vi "DefaultFromINI.vi"(8 "error in (no error)":errorcluster, 11 "NhRegenGridSim":refnum<class "NHRGridSim.lvclass">) -> (0 "error out":errorcluster, 3 "NhRegenGridSim":refnum<class "NHRGridSim.lvclass">)   [LabVIEW 2018, in "AcPwrPlugins.lvlib" / "NHRGridSim.lvclass"]
doc: "This VI reads the properties from the INI file and puts them into the LabVIEW class for further use."
uses:
  NHRGridSim.lvclass
  C:/Program Files (x86)/National Instruments/LabVIEW 2018/user.lib/NIST/BaseClasses/BasePlugin_class/BasePlugin.lvclass
  C:/Projects/SmartGrid/ICDAS/NistPluggableModules/AcPwr/AcPwrPlugins/AcPwrBaseClass/AcPwrBase.lvclass
  Measurements.ctl
  TypeDefs/MeasurementType.ctl
  TypeDefs/Device(s)Settings.ctl
  TypeDefs/Modules.ctl
  <userlib>/NIST/BaseClasses/BasePlugin_class/BasePlugin.lvclass/BasePlugin.ctl
  <userlib>/NIST/BaseClasses/BasePlugin_class/Accessors/Read PluginIniFilePath.vi
  AcPwrBaseClass/AcPwrBase.lvclass
  <vilib>/Utility/config.llb/NI_LVConfig.lvlib
  TestClass/Test.lvclass
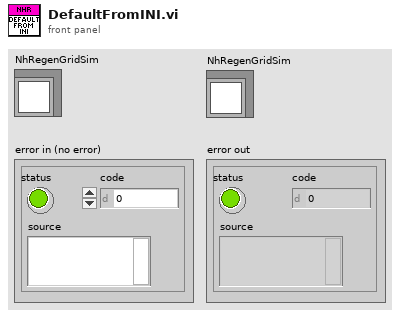
[diagram p1: front panel]
types:
  T1 = typedef "AcPwrPlugins.lvlib/NHRGridSim.lvclass/Device(s)Settings.ctl" = cluster{"MeasName":string, "Modules":T2}
  T2 = typedef "AcPwrPlugins.lvlib/NHRGridSim.lvclass/Modules.ctl" = cluster{"Measurement":cluster{"ApertureLength (s)":dbl, "NumberOfSamples":u32}, "Ranges":cluster{"Irange (A)":dbl, "Vrange (V)":dbl}, "Mode":u8, "Handle":string, "FreqOut (Hz)":dbl, "Connected":bool, "btnIdQuery":bool, "btnReset":bool, "Initialize Timeout ( ms)":u32, "Phase (0: All)":i32, "WatchDog":cluster{"Enable WatchDog":bool, "Robust WatchDog":bool, "Watchdog Interval (s)":dbl}, "Safety Limits":cluster{"Min Voltage (V)":dbl, "Min Voltage Time (s)":dbl, "Max Voltage (V)":dbl, "MaxVoltage Time (s)":dbl, "Max Source Amps (A)":dbl, "Max Source Amps Time (s)":dbl, "Max Sink Amps (A)":dbl, "Max Sink Amps Time (s)":dbl, "Max Source Power (W)":dbl, "Max Source Power Time (s)":dbl, "Max Sink Power (W)":dbl, "Max Sink Power Time (s)":dbl, "Peak Voltage (V)":dbl, "Peak Voltage Enable":bool, "Peak Amps (A)":dbl, "Peak Amps Enable":bool}, "Phases":cluster{"Pout (W)":dbl, "Iout (A)":dbl, "PhaseAngle":dbl, "Vout (V)":dbl, "Phase Name":string}[], "Regulation Gain":dbl, "ChangeOntheFly":bool, "Synchronize Output \nto Phase":bool, "Slew Rate":cluster{"Voltage Slew (Volts/s)":dbl, "Phase Angle (Degrees/s)":dbl}}[]
  T3 = typedef "AcPwrPlugins.lvlib/NHRGridSim.lvclass/Measurements.ctl" = cluster{"Handle":string, "Name":string, "Enabled ":bool, "Measurement Value":dbl, "Phase ":i32, "Measurement Type ":T4}[]
  T4 = typedef "AcPwrPlugins.lvlib/NHRGridSim.lvclass/MeasurementType.ctl" = enum16{"Average Current", "Average Voltage"}
  T5 = typedef "NI_LVConfig.lvlib/Config Data RefNum.ctl" = refnum<k1>
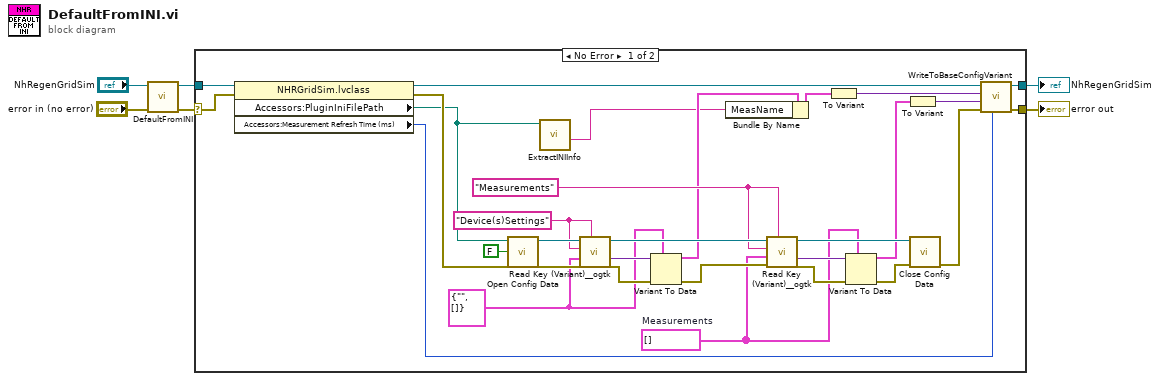
[diagram p0: block diagram]
diagram:
  n1 = call-parent "DefaultFromINI.vi"("error in (no error)"="error in (no error)", "AcPwrBase"="NhRegenGridSim") -> ("error out"=w1:errorcluster, "AcPwrBase"=w4:refnum<class "NHRGridSim.lvclass">)  [unwired: 8 in]
  n2 = case shown="No Error" w1 {
    selector: w1 -> [w29 w37]
    tunnel: w4 -> [w36 w38]
    tunnel: [w12 w38] -> w6
    tunnel: [w18 w37] -> w5
    frame No Error {
      w10 = T1 {"MeasName"="", "Modules"=[]} ("Device(s)Settings")
      w20 = T3 []  # Measurements
      w21 = "Measurements" ("section")
      w30 = "Device(s)Settings" ("section")
      n3 = property class="NHRGridSim.lvclass"(reference=w36, error in=w29) -> (reference out=w13:refnum<class "NHRGridSim.lvclass">, error out=w28:errorcluster, "Accessors:PluginIniFilePath"=w8:path, "Accessors:Measurement Refresh Time (ms)"=w11:u32)
      n4 = call <vilib>:"Open Config Data.vi"("error in (no error)"=w28, "create file if necessary (T)"=FALSE, "configuration file path"=w8) -> ("error out"=w33:errorcluster, "refnum"=w34:T5)  [unwired: 6 in, 1 out]
      n5 = call "ExtractINIInfo.vi"("INI File Path"=w8) -> ("Plugin Name"=w7:string)  [unwired: 8 in, 2 out]
      n6 = call <userlib>:"Read Key (Variant)__ogtk.vi"("section"=w30, "error in (no error)"=w33, "type"=w10, "key (optional)"=w30, "refnum"=w34) -> ("error out"=w31:errorcluster, "key-value"=w32:variant, "refnum out"=w25:T5)  [unwired: 3 in, 1 out]
      n7 = Variant To Data(error in=w31, type=w10, Variant=w32) -> (data=w14:T1, error out=w22:errorcluster)
      n8 = Bundle By Name(cluster=w14, "MeasName"=w7) -> (w9:T1)
      n9 = call <userlib>:"Read Key (Variant)__ogtk.vi"("section"=w21, "error in (no error)"=w22, "type"=w20, "key (optional)"=w21, "refnum"=w25) -> ("error out"=w27:errorcluster, "key-value"=w26:variant, "refnum out"=w24:T5)  [unwired: 3 in, 1 out]
      n10 = To Variant(anything=w9) -> (Variant=w16:variant)
      n11 = Variant To Data(error in=w27, type=w20, Variant=w26) -> (data=w15:T3, error out=w23:errorcluster)
      n12 = To Variant(anything=w15) -> (Variant=w17:variant)
      n13 = call <vilib>:"Close Config Data.vi"("error in (no error)"=w23, "refnum"=w24) -> ("error out"=w19:errorcluster)  [unwired: 8 in, 1 out]
      n14 = call "WriteToBaseConfigVariant.vi"("Measurement RefreshTime (ms)"=w11, "error in (no error)"=w19, "Meas"=w17, "Config"=w16, "NHRGridSim in"=w13) -> ("error out"=w18:errorcluster, "NHRGridSim out"=w12:refnum<class "NHRGridSim.lvclass">)  [unwired: 5 in]
    }
    frame Error {
    }
  }
  "error out" <- w5
  "NhRegenGridSim" <- w6
